vi "Set Control File Attributes.vi"(8 "error in (no error)":errorcluster, 10 "package attributes":T1={"Package Name"="", "Display name"="", "Version"="", "Display version"="", "Synopsis"="", "Description"="", "Maintainer"="", "Maintainer email address"="", "Category"="", "Homepage"="", "Release notes"="", "Depends"=[], "Recommends"=[], "Suggests"=[], "Conflicts"=[], "Provides"=[], "Replaces"=[], "Supplements"=[], "Enhances"=[], "Product"=FALSE, "User visible"=FALSE, "Installed size (KB)"=0, "Package filesize (bytes)"=0, "Architecture"="", "Agent"="file", "MD5Checksum"=""}, 11 "control file refnum in":refnum<file>) -> (0 "error out":errorcluster, 3 "control file refnum out":refnum<file>)   [LabVIEW 2014, in "NIPM_API.lvlib"]
doc: "Modifies the package attributes in an unpacked package's control file.\n\nINPUT(s)\n<B>Control file refnum in</B>: This is a file refnum from an unpacked package's control file. Use the Open/Create/Replace File function to open a control file and pass its file refnum to this VI.\n\n<B>Package attributes</B>: This VI writes these package attributes and values to the control file.\n\nOUTPUT(s)\n<B>Control file refnum out</B>: Passes the control file refnum out of this VI.\n\nDETAILS\nFor additional details on the control file attributes, refer to the following link:\nhttp://www.ni.com/documentation/en/ni-package-manager/latest/manual/control-file-attributes/"
uses:
  NIPM_API.lvlib
  _support/package attributes.ctl
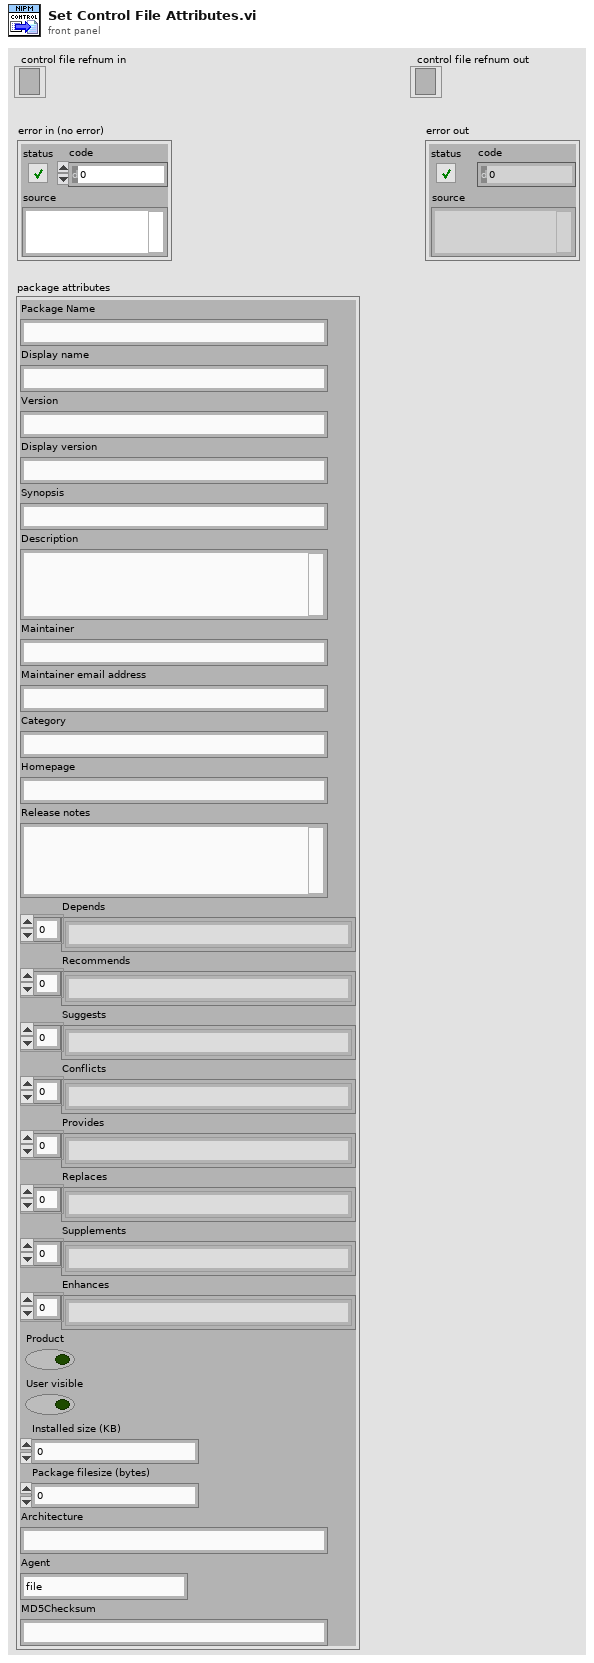
[diagram p1: front panel]
types:
  T1 = typedef "NIPM_API.lvlib/package attributes.ctl" = cluster{"Package Name":string, "Display name":string, "Version":string, "Display version":string, "Synopsis":string, "Description":string, "Maintainer":string, "Maintainer email address":string, "Category":string, "Homepage":string, "Release notes":string, "Depends":string[], "Recommends":string[], "Suggests":string[], "Conflicts":string[], "Provides":string[], "Replaces":string[], "Supplements":string[], "Enhances":string[], "Product":bool, "User visible":bool, "Installed size (KB)":u64, "Package filesize (bytes)":u64, "Architecture":string, "Agent":string, "MD5Checksum":string}
  T2 = enum16{"open", "replace", "create", "open or create", "replace or create", "replace or create with confirmation"}
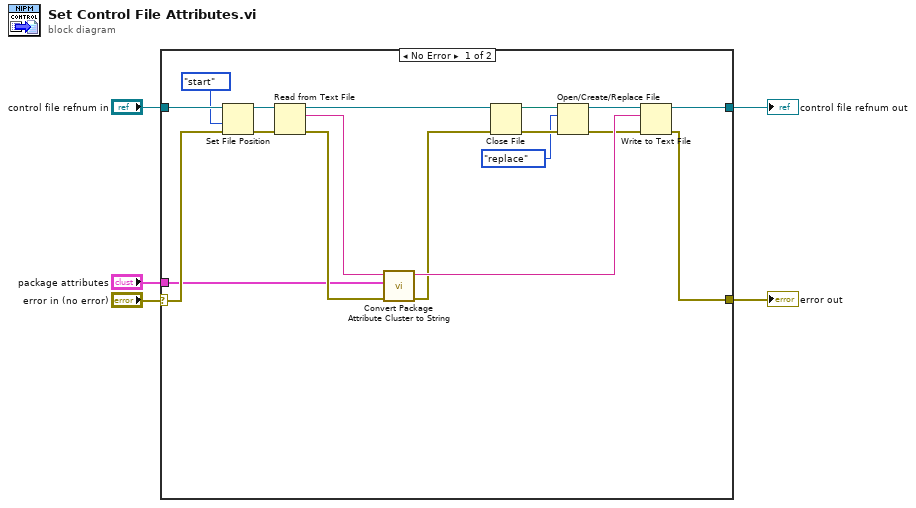
[diagram p0: block diagram]
diagram:
  n1 = case shown="No Error" "error in (no error)" {
    selector: "error in (no error)" -> [w18 w25]
    tunnel: "control file refnum in" -> [w15 w24]
    tunnel: [w19 w24] -> w4
    tunnel: [w20 w25] -> w2
    tunnel: "package attributes" -> [w12 _]
    frame No Error {
      n2 = Set File Position(refnum=w15, from (0:start)=enum16{"start", "end", "current"}."start", error in=w18) -> (refnum out=w14:refnum<file>, error out=w16:errorcluster)  [unwired: 1 in]
      n3 = Read from Text File(file (use dialog)=w14, error in=w16) -> (refnum out=w22:refnum<file>, text=w23:string, error out=w17:errorcluster)  [unwired: 2 in, 1 out]
      n4 = call "Convert Package Attribute Cluster to String.vi"("error in (no error)"=w17, "package attributes"=w12, "initial package attributes string"=w23) -> ("error out"=w9:errorcluster, "package attributes string out"=w21:string)  [unwired: 7 in]
      n5 = Close File(refnum=w22, error in=w9) -> (path=w11:path, error out=w8:errorcluster)
      n6 = Open/Create/Replace File(file path (use dialog)=w11, error in=w8, operation (0:open)=T2."replace") -> (refnum out=w10:refnum<file>, error out=w7:errorcluster)  [unwired: 3 in, 1 out]
      n7 = Write to Text File(file (use dialog)=w10, text=w21, error in=w7) -> (refnum out=w19:refnum<file>, error out=w20:errorcluster)  [unwired: 1 in, 1 out]
    }
    frame Error {
    }
  }
  "control file refnum out" <- w4
  "error out" <- w2
